vi "Read Task Type.vi"(8 "error in (no error)":errorcluster, 11 "Task Ancestor in":refnum<class "Task Ancestor.lvclass">) -> (0 "error out":errorcluster, 2 "Task ID":i64, 3 "Task Ancestor out":refnum<class "Task Ancestor.lvclass">)   [LabVIEW 2024, in "Task Ancestor.lvclass"]
uses:
  Task Ancestor.lvclass
  Task Ancestor.lvclass/Task Ancestor.ctl
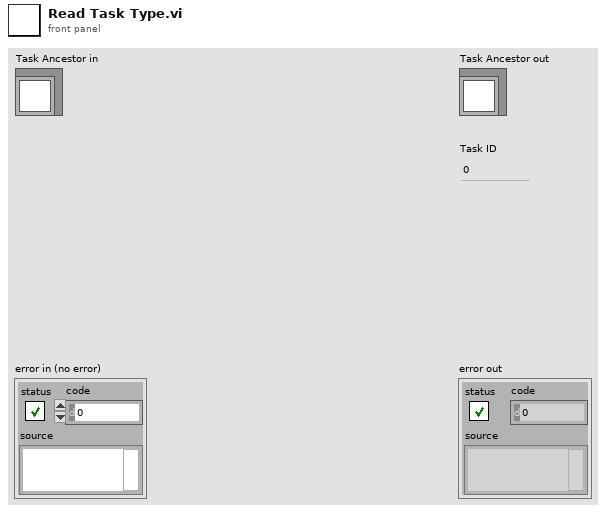
[diagram p1: front panel]
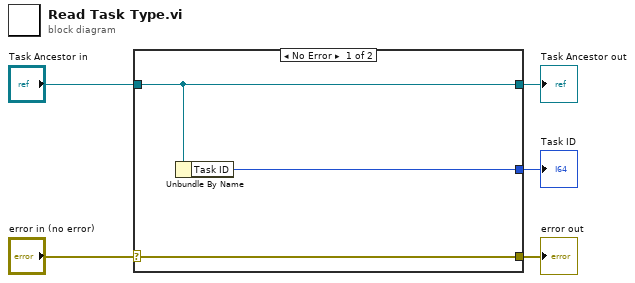
[diagram p0: block diagram]
diagram:
  n1 = case shown="No Error" "error in (no error)" {
    selector: "error in (no error)" -> [w8 w9]
    tunnel: [w8 w9] -> w4
    tunnel: [w7 w10] -> w2
    tunnel: "Task Ancestor in" -> [w7 w10]
    tunnel: [w6 _] -> w1
    frame No Error {
      n2 = Unbundle By Name(w7) -> ("Task ID"=w6:i64)
    }
    frame Error {
    }
  }
  "error out" <- w4
  "Task Ancestor out" <- w2
  "Task ID" <- w1
